vi "VISA Command.vi"(7 "Wait (ms)":u32=400, 8 "error in (no error)":errorcluster, 10 "Command":string, 11 "VISA resource name":refnum<visa-resource-name>) -> (0 "error out":errorcluster, 2 "read buffer":string, 3 "VISA resource name out":refnum<visa-resource-name>)   [LabVIEW 2019, in "IDEX.lvlib"]
uses:
  IDEX.lvlib
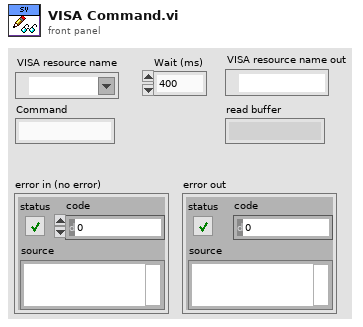
[diagram p1: front panel]
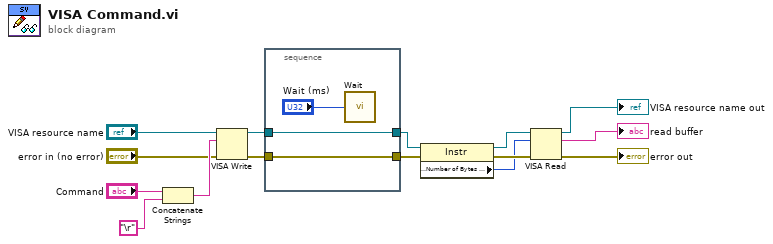
[diagram p0: block diagram]
diagram:
  n1 = Concatenate Strings("Command", "\r") -> (w10:string)
  n2 = VISA Write(VISA resource name="VISA resource name", write buffer=w10, error in (no error)="error in (no error)") -> (VISA resource name out=w13:refnum<visa-resource-name>, error out=w15:errorcluster)  [unwired: 1 out]
  n3 = stacked-sequence {
    tunnel: w15 -> [w18]
    tunnel: [w18] -> w14
    tunnel: w13 -> [w17]
    tunnel: [w17] -> w12
    frame #0 {
      n4 = call "Wait"("Count(mSec)"="Wait (ms)") -> ()  [unwired: 1 out]
    }
  }
  n5 = property class="Instr"(reference=w12, error in=w14) -> (reference out=w11:refnum<visa-resource-name>, error out=w9:errorcluster, "Serial Settings:Number of Bytes at Serial Port"=w8:u32)
  n6 = VISA Read(VISA resource name=w11, byte count=w8, error in (no error)=w9) -> (VISA resource name out=→"VISA resource name out":refnum<visa-resource-name>, read buffer=→"read buffer":string, error out=→"error out":errorcluster)  [unwired: 1 out]
